vi "Control de Temperatura Max-Min.vi"() -> ()   [LabVIEW 2019]
panel:
  in  "Decremento T":dbl(knob) scale=0.0..10.0
  in  "Incremento T":dbl(knob) scale=0.0..10.0
  out "Decremento":bool
  out "Incremento":bool
  in  "Selector":bool
  in  "RATA DE T (°C/Seg)":dbl(knob) scale=0.0..10.0
  in  "Temp Mín":dbl
  in  "Temp Máx":dbl
  out "Sensor de Temperatura °C":dbl(slide) scale=0.0..200.0
  # "DECREMENTAR"
  # "INCREMENTAR"
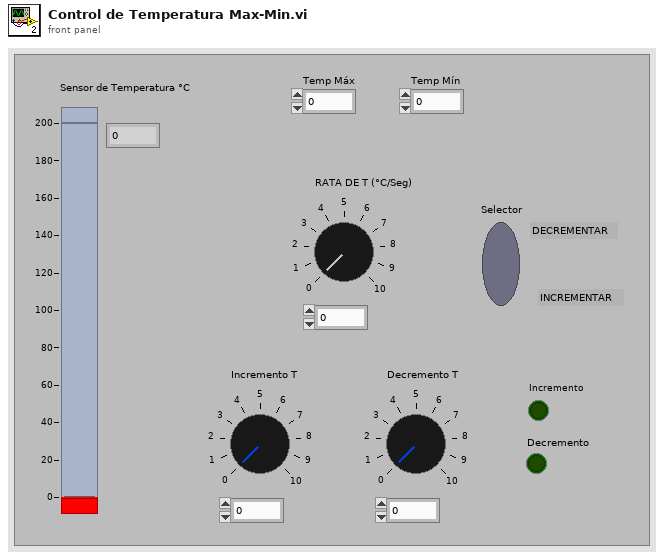
[diagram p1: front panel]
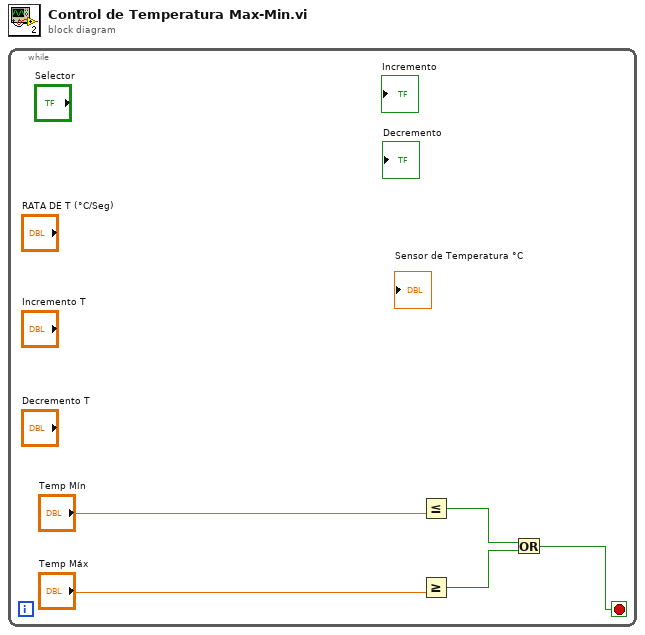
[diagram p0: block diagram]
diagram:
  n1 = while {
    stop <- w5 stop-if-true
    n2 = Less Or Equal?(y="Temp Mín") -> (x <= y?=w2:bool)  [unwired: 1 in]
    n3 = Greater Or Equal?(y="Temp Máx") -> (x >= y?=w3:bool)  [unwired: 1 in]
    n4 = Or(x=w2, y=w3) -> (x .or. y?=w5:bool)
  }
